vi "IS Epoch Time.vi"(11 "Stream Time (optional)":timestamp=timestamp(1451714400 s since 1904-01-01)) -> (3 "Time (epoch)":dbl format="%#_15f")   [LabVIEW 2013]
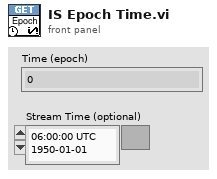
[diagram p1: front panel]
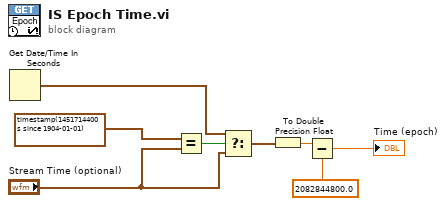
[diagram p0: block diagram]
diagram:
  n1 = Get Date/Time In Seconds() -> (seconds since 1Jan1904=w2:timestamp)
  n2 = Equal?(x=timestamp(1451714400 s since 1904-01-01) ("Stream Time (optional)"), y="Stream Time (optional)") -> (x = y?=w4:bool)
  n3 = Select(t=w2, s=w4, f="Stream Time (optional)") -> (s? t:f=w1:timestamp)
  n4 = To Double Precision Float(number=w1) -> (double precision float=w6:dbl)
  n5 = Subtract(x=w6, y=2082844800.0) -> (x-y=→"Time (epoch)":dbl)
